vi "Parse-attribute.vi"(8 "error in (no error)":errorcluster, 10 "String in":string, 11 "Attribute-XML in":refnum<class "Attribute-XML.lvclass">) -> (0 "error out":errorcluster, 1 "Valid attribute?":bool, 2 "Remaining string":string, 3 "Attribute-XML out":refnum<class "Attribute-XML.lvclass">)   [LabVIEW 2013, in "MaterialCharacterization.lvlib" / "Attribute-XML.lvclass"]
uses:
  Attribute-XML.lvclass
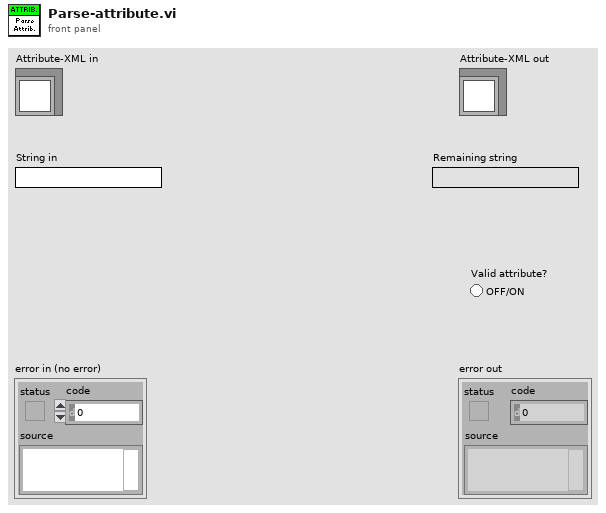
[diagram p1: front panel]
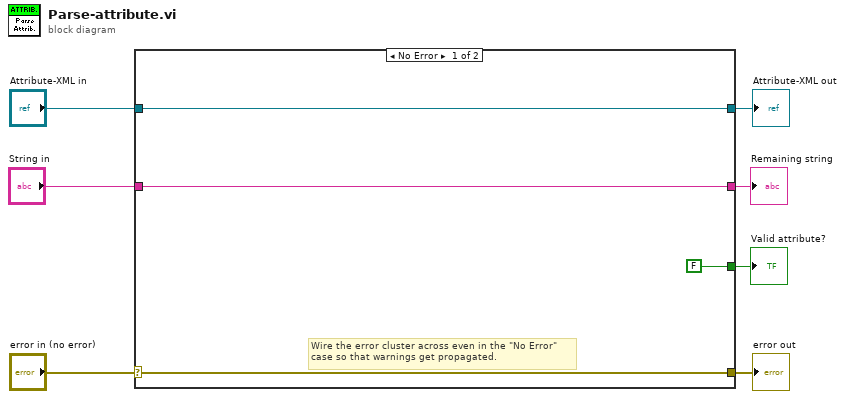
[diagram p0: block diagram]
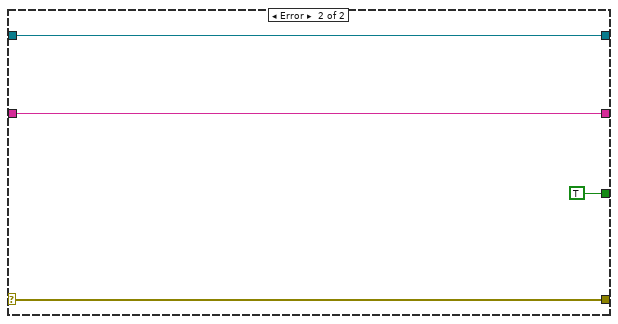
[diagram p2: hidden frame]
diagram:
  n1 = case shown="No Error" "error in (no error)" {
    selector: "error in (no error)" -> [w10 w15]
    tunnel: [w10 w15] -> w6
    tunnel: [w11 w14] -> w4
    tunnel: "Attribute-XML in" -> [w11 w14]
    tunnel: "String in" -> [w9 w12]
    tunnel: [w9 w12] -> w2
    tunnel: [FALSE TRUE] -> w1
    frame No Error {
      # "Wire the error cluster across even in the \"No Error\"\ncase so that warnings get propagated."
    }
    frame Error {
    }
  }
  "error out" <- w6
  "Attribute-XML out" <- w4
  "Remaining string" <- w2
  "Valid attribute?" <- w1
